vi "Select Channels.vi"(8 "error in (no error)":errorcluster, 11 "Node Ptr":T1 format="%.0x") -> (0 "error out":errorcluster, 3 "Node Ptr":T1[](array[typedef]) format="%.0x")   [LabVIEW 2013]
uses:
  <vilib>/NI Veristand/Custom Device Tools/Custom Device Utility Library/Custom Device Utility Library.lvlib
  <vilib>/NI Veristand/Custom Device API/Custom Device API.lvlib
  <vilib>/NI Veristand/Custom Device API/Set Item Property (String Array).vi
  <vilib>/NI Veristand/Custom Device API/Custom Device Item Ref.ctl
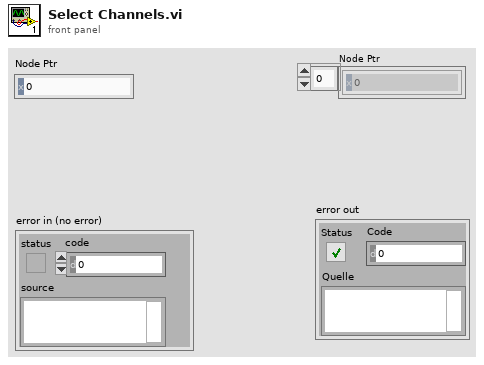
[diagram p1: front panel]
types:
  T1 = typedef "Custom Device API.lvlib/Custom Device Item Ref.ctl" = u64
  T2 = typedef "Custom Device API.lvlib/Custom Device Item Info.ctl" = cluster{"Name":string, "Is Channel":bool, "GUID":string, "Is Waveform":bool}
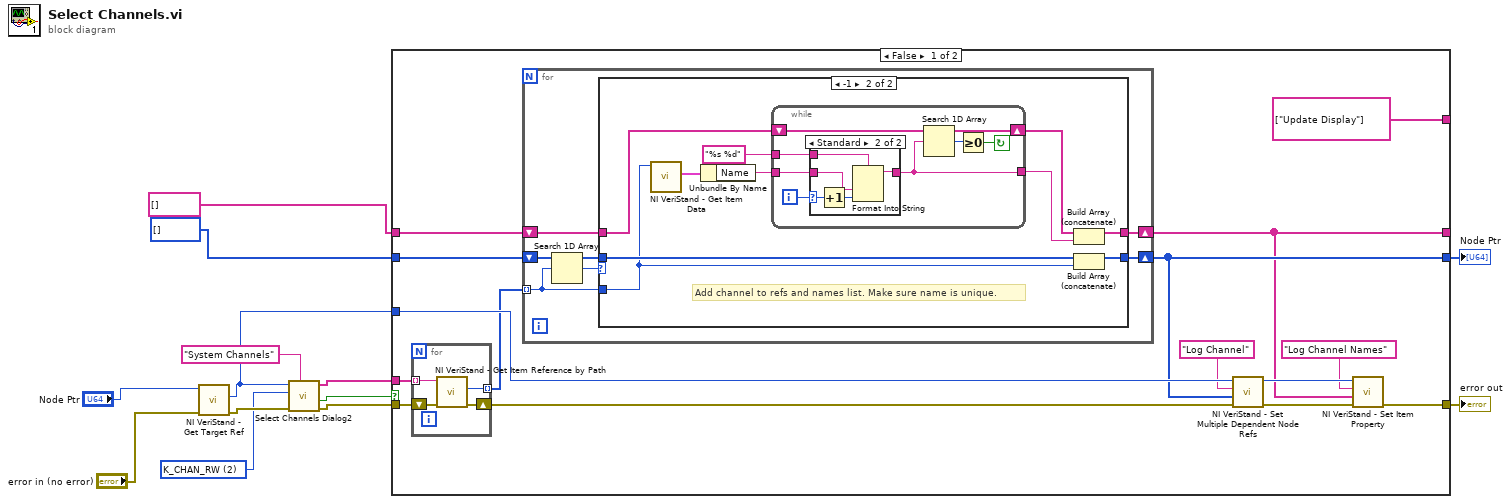
[diagram p0: block diagram]
diagram:
  w10 = u8 2 items=["K_CHAN_R", "K_CHAN_W", "K_CHAN_RW", "K_CHAN_VOLT", "K_CHAN_FAULT", "K_ALL", "K_CUSTOM"] ("Filter")
  n1 = call <vilib>:"NI VeriStand - Get Target Ref.vi"("error in"="error in (no error)", "Item Ref in"="Node Ptr") -> ("error out"=w11:errorcluster, "Target Ref"=w6:T1)  [unwired: 6 in, 2 out]
  n2 = call "Select Channels Dialog2.vi"("Channel Label"="System Channels", "error in (no error)"=w11, "Filter"=w10, "Start Item Ref"=w6) -> ("error out"=w9:errorcluster, "Canceled"=w7:bool, "Channels"=w8:string[])  [unwired: 2 in, 3 out]
  n3 = case shown="False" w7 {
    tunnel: T1[] [] ("Selected Channel Refs") -> [w28 w66]
    tunnel: w9 -> [w17 w65]
    tunnel: w8 -> [w16 _]
    tunnel: [w24 w66] -> w1
    tunnel: [w18 w65] -> w2
    tunnel: w6 -> [w25 _]
    tunnel: [string[] ["Update Display"] _] -> _
    tunnel: string[] [] -> [w26 w64]
    tunnel: [w19 w64] -> _
    frame False {
      n4 = for {
        shift-right: [w31] -> w14
        shift-left: w17 -> [w32]
        tunnel: w16 -> [w30] mode=indexing
        tunnel: [w29] -> w15 mode=indexing
        n5 = call <vilib>:"NI VeriStand - Get Item Reference by Path.vi"("error in (no error)"=w32, "Item Path in"=w30) -> ("error out"=w31:errorcluster, "Item Ref"=w29:T1)  [unwired: 6 in, 2 out]
      }
      n6 = for {
        shift-right: [w36] -> w24
        shift-left: w28 -> [w37]
        shift-right: [w34] -> w19
        shift-left: w26 -> [w35]
        tunnel: w15 -> [w33] mode=indexing
        n7 = Search 1D Array(1D array=w37, element=w33) -> (index of element=w38:i32)  [unwired: 1 out]
        n8 = case shown="-1" w38 {
          tunnel: w37 -> [w40 w50]
          tunnel: [w40 w49] -> w36
          tunnel: w33 -> [_ w48]
          tunnel: w35 -> [w39 w43]
          tunnel: [w39 w46] -> w34
          frame Default {
            # "Channel already selected for logging. Don't add to refs or names list."
          }
          frame -1 {
            # "Add channel to refs and names list. Make sure name is unique."
            n9 = call <vilib>:"NI VeriStand - Get Item Data.vi"("Item Ref in"=w48) -> ("Item Info"=w47:T2)  [unwired: 1 in, 9 out]
            n10 = Unbundle By Name(w47) -> ("Name"=w42:string)
            n11 = while {
              shift-right: [w55] -> w44
              shift-left: w43 -> [w55]
              tunnel: w42 -> [w56]
              tunnel: [w52] -> w41
              tunnel: "%s %d" ("format string") -> [w51]
              i -> [w57]
              stop <- w53 continue-if-true
              n12 = case shown="Standard" w57 {
                selector: w57 -> [_ w61]
                tunnel: w56 -> [w58 w59]
                tunnel: [w58 w63] -> w52
                tunnel: w51 -> [_ w62]
                frame 0 {
                }
                frame Default {
                  n13 = Increment(x=w61) -> (x+1=w60:i32)
                  n14 = Format Into String(format string=w62, w59, w60) -> (resulting string=w63:string)  [unwired: 2 in, 1 out]
                }
              }
              n15 = Search 1D Array(1D array=w55, element=w52) -> (index of element=w54:i32)  [unwired: 1 out]
              n16 = Greater Or Equal To 0?(x=w54) -> (x >= 0?=w53:bool)
            }
            n17 = Build Array (concatenate)(w44, w41) -> (w46:string[])
            n18 = Build Array (concatenate)(w50, w48) -> (w49:T1[])
          }
        }
      }
      n19 = call <vilib>:"NI VeriStand - Set Multiple Dependent Node Refs.vi"("error in (no error)"=w14, "Dependent Node Refs"=w24, "Base Property Name"="Log Channel" ("Property Name"), "Item Ref in"=w25) -> ("error out"=w21:errorcluster, "Item Ref out"=w22:T1)  [unwired: 6 in]
      n20 = call-poly <vilib>:"NI VeriStand - Set Item Property.vi"("error in (no error)"=w21, "Value"=w19, "Property Name"="Log Channel Names", "Item Ref in"=w22) -> ("error out"=w18:errorcluster)  [unwired: 5 in, 2 out]
    }
    frame True {
      # "User canceled out of the dialog."
    }
  }
  "error out" <- w2
  "Node Ptr" <- w1
